vi "Enviar datos.vi"(7 "Proviene de?":enum16{"Contador", "Generador funciones"}(ring), 8 "error in (no error)":errorcluster, 9 "Dato":string, 10 "Path":path, 11 "Guardar Tipo CSV in":refnum<class "Guardar Tipo CSV.lvclass">) -> (0 "error out":errorcluster, 3 "Guardar Tipo CSV out":refnum<class "Guardar Tipo CSV.lvclass">)   [LabVIEW 2020, in "Guardar Tipo CSV.lvlib" / "Guardar Tipo CSV.lvclass"]
uses:
  Guardar Tipo CSV.lvclass
  Guardar Tipo CSV.lvclass/Guardar Tipo CSV.ctl
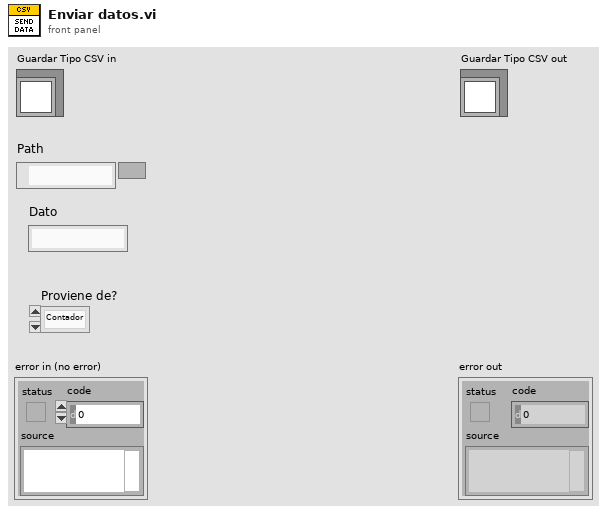
[diagram p1: front panel]
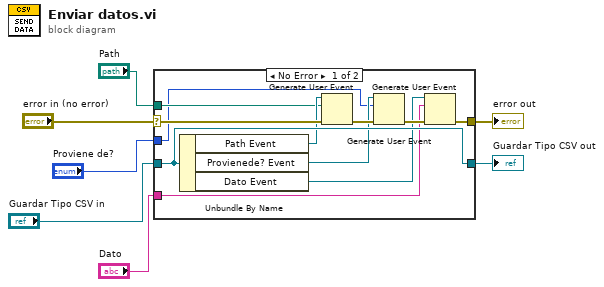
[diagram p0: block diagram]
diagram:
  n1 = case shown="No Error" "error in (no error)" {
    selector: "error in (no error)" -> [w14 w20]
    tunnel: [w17 w20] -> w6
    tunnel: [w18 w19] -> w4
    tunnel: "Guardar Tipo CSV in" -> [w18 w19]
    tunnel: "Path" -> [w12 _]
    tunnel: "Proviene de?" -> [w10 _]
    tunnel: "Dato" -> [w8 _]
    frame No Error {
      n2 = Unbundle By Name(w18) -> ("Path Event"=w13:refnum<user-event>, "Provienede? Event"=w11:refnum<user-event>, "Dato Event"=w9:refnum<user-event>)
      n3 = Generate User Event(user event=w13, event data cluster=w12, error in=w14) -> (error out=w15:errorcluster)  [unwired: 1 in, 1 out]
      n4 = Generate User Event(user event=w11, event data cluster=w10, error in=w15) -> (error out=w16:errorcluster)  [unwired: 1 in, 1 out]
      n5 = Generate User Event(user event=w9, event data cluster=w8, error in=w16) -> (error out=w17:errorcluster)  [unwired: 1 in, 1 out]
    }
    frame Error {
    }
  }
  "error out" <- w6
  "Guardar Tipo CSV out" <- w4
